vi "Init.vi"(8 "error in (no error)":errorcluster, 11 "IV in":refnum<class "IV.lvclass">) -> (0 "error out":errorcluster, 2 "File Path":path, 3 "IV out":refnum<class "IV.lvclass">)   [LabVIEW 2021, in "IV.lvclass"]
uses:
  IV.lvclass
  Libraries/Instruments/Results/Acquired Result/Acquired Result.lvclass
  Libraries/File/File Class/File.lvclass/File.ctl
  Libraries/File/File Class/Write File Prefix.vi
  Libraries/File/File Class/Write Include time.vi
  Libraries/File/File Class/File.lvclass
  Libraries/Instruments/Instrument Driver/Instrument Driver.lvclass
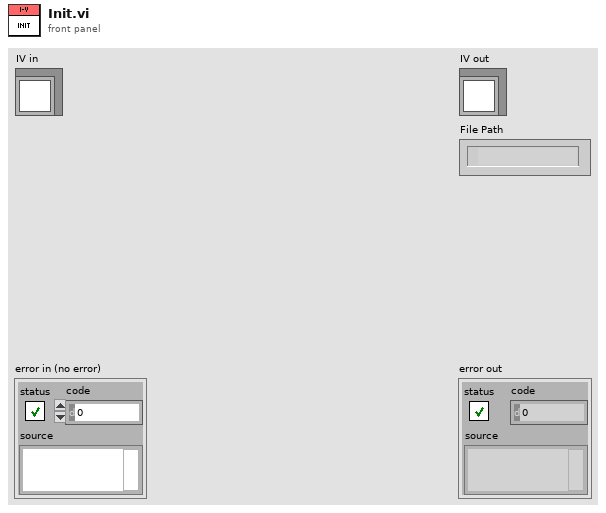
[diagram p1: front panel]
types:
  T1 = typedef "IV Config.ctl" = cluster{"Start current":dbl, "End current":dbl, "Current step":dbl, "Step time":dbl}
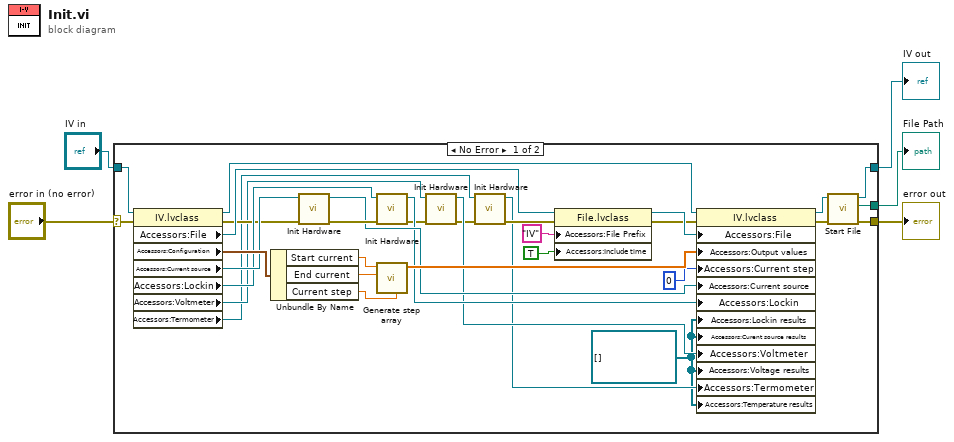
[diagram p0: block diagram]
diagram:
  n1 = case shown="No Error" "error in (no error)" {
    selector: "error in (no error)" -> [w38 w40]
    tunnel: [w31 w40] -> w4
    tunnel: [w33 w39] -> w2
    tunnel: "IV in" -> [w26 w39]
    tunnel: [w30 _] -> w1
    frame No Error {
      w6 = refnum<class "Acquired Result.lvclass">[] [] ("Lockin results")
      n2 = property class="IV.lvclass"(reference=w26, error in=w38) -> (reference out=w25:refnum<class "IV.lvclass">, error out=w17:errorcluster, "Accessors:File"=w24:refnum<class "File.lvclass">, "Accessors:Configuration"=w23:T1, "Accessors:Current source "=w19:refnum<class "Instrument Driver.lvclass">, "Accessors:Lockin"=w18:refnum<class "Instrument Driver.lvclass">, "Accessors:Voltmeter"=w12:refnum<class "Instrument Driver.lvclass">, "Accessors:Termometer"=w10:refnum<class "Instrument Driver.lvclass">)
      n3 = Unbundle By Name(w23) -> ("Start current"=w29:dbl, "End current"=w28:dbl, "Current step"=w27:dbl)
      n4 = call-dynamic "Init Hardware.vi"("error in (no error)"=w17, "Instrument Driver in"=w19) -> ("error out"=w16:errorcluster, "Instrument Driver out"=w15:refnum<class "Instrument Driver.lvclass">)  [unwired: 8 in]
      n5 = call-dynamic "Init Hardware.vi"("error in (no error)"=w16, "Instrument Driver in"=w18) -> ("error out"=w13:errorcluster, "Instrument Driver out"=w14:refnum<class "Instrument Driver.lvclass">)  [unwired: 8 in]
      n6 = call "Generate step array.vi"("Step"=w27, "End"=w28, "Start"=w29) -> ("Steps"=w22:dbl[])  [unwired: 8 in]
      n7 = call-dynamic "Init Hardware.vi"("error in (no error)"=w13, "Instrument Driver in"=w12) -> ("error out"=w9:errorcluster, "Instrument Driver out"=w11:refnum<class "Instrument Driver.lvclass">)  [unwired: 8 in]
      n8 = call-dynamic "Init Hardware.vi"("error in (no error)"=w9, "Instrument Driver in"=w10) -> ("error out"=w8:errorcluster, "Instrument Driver out"=w7:refnum<class "Instrument Driver.lvclass">)  [unwired: 8 in]
      n9 = property class="File.lvclass"(reference=w24, error in=w8, "Accessors:File Prefix"="IV" ("File Prefix"), "Accessors:Include time"=TRUE ("Include time")) -> (reference out=w35:refnum<class "File.lvclass">, error out=w20:errorcluster)
      n10 = property class="IV.lvclass"(reference=w25, error in=w20, "Accessors:File"=w35, "Accessors:Output values"=w22, "Accessors:Current step"=0 ("Current step"), "Accessors:Current source "=w15, "Accessors:Lockin"=w14, "Accessors:Lockin results"=w6, "Accessors:Curent source results"=w6, "Accessors:Voltmeter"=w11, "Accessors:Voltage results"=w6, "Accessors:Termometer"=w7, "Accessors:Temperature results"=w6) -> (reference out=w34:refnum<class "IV.lvclass">, error out=w32:errorcluster)
      n11 = call-dynamic "Start File.vi"("error in (no error)"=w32, "Pulse Echo in"=w34) -> ("error out"=w31:errorcluster, "File Path"=w30:path, "Pulse Echo out"=w33:refnum<class "IV.lvclass">)  [unwired: 7 in]
    }
    frame Error {
    }
  }
  "error out" <- w4
  "IV out" <- w2
  "File Path" <- w1
